vi "DAC_example.vi"() -> ()   [LabVIEW 2009]
panel:
  out "ACV Result":dbl[](array[numeric]) format="%.2e"
  out "Frequency Result":dbl[](array[numeric]) format="%.2e"
  out "VISA/Instrument Errors":errorcluster
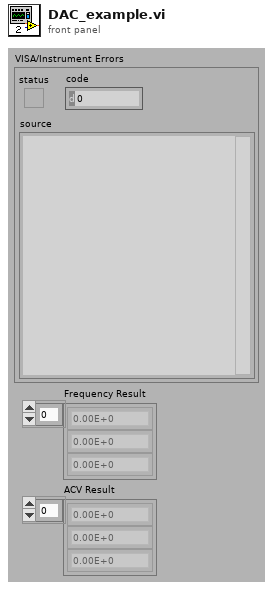
[diagram p1: front panel]
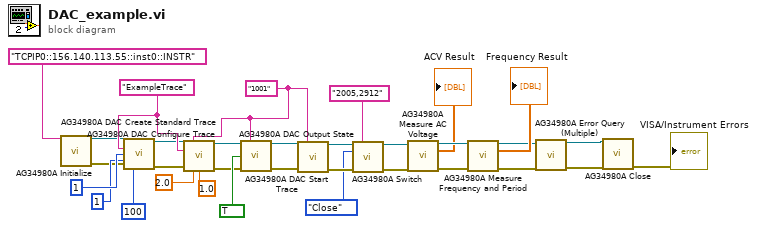
[diagram p0: block diagram]
diagram:
  w17 = "1001"
  w26 = "ExampleTrace"
  n1 = call "AG34980A Initialize.vi"("VISA resource name"="TCPIP0::156.140.113.55::inst0::INSTR") -> ("VISA session"=w25:refnum<visa-resource-name>, "error out"=w24:errorcluster)  [unwired: 13 in]
  n2 = call "AG34980A DAC Create Standard Trace.vi"("VISA resource name"=w25, "Trace Name"=w26, "Slot (1)"=1, "Trace Type"=1, "error in (no error)"=w24, "Num Points (1000)"=100) -> ("VISA resource name out"=w23:refnum<visa-resource-name>, "error out"=w22:errorcluster)  [unwired: 8 in]
  n3 = call "AG34980A DAC Configure Trace.vi"("VISA resource name"=w23, "Channel List"=w17, "Trace Name"=w26, "error in (no error)"=w22, "Gain (1)"=2.0, "Offset (0)"=1.0) -> ("VISA resource name out"=w21:refnum<visa-resource-name>, "error out"=w20:errorcluster)  [unwired: 8 in]
  n4 = call "AG34980A DAC Output State.vi"("VISA resource name"=w21, "Channel List"=w17, "Output State (F:Off)"=TRUE, "error in (no error)"=w20) -> ("VISA resource name out"=w19:refnum<visa-resource-name>, "error out"=w18:errorcluster)  [unwired: 10 in]
  n5 = call "AG34980A DAC Start Trace.vi"("VISA resource name"=w19, "Channel List"=w17, "error in (no error)"=w18) -> ("VISA resource name out"=w8:refnum<visa-resource-name>, "error out"=w7:errorcluster)  [unwired: 11 in]
  n6 = call "AG34980A Switch.vi"("VISA resource name"=w8, "Channel List"="2005,2912", "Open/Close (0:Close)"=enum16{"Close", "Open"}."Close", "error in (no error)"=w7) -> ("VISA resource name out"=w6:refnum<visa-resource-name>, "error out"=w5:errorcluster)  [unwired: 9 in, 1 out]
  n7 = call "AG34980A Measure AC Voltage.vi"("VISA resource name"=w6, "error in (no error)"=w5) -> ("VISA resource name out"=w13:refnum<visa-resource-name>, "Output Array"=→"ACV Result":dbl[], "error out"=w14:errorcluster)  [unwired: 11 in]
  n8 = call "AG34980A Measure Frequency and Period.vi"("VISA resource name"=w13, "error in (no error)"=w14) -> ("VISA resource name out"=w10:refnum<visa-resource-name>, "Output Array"=→"Frequency Result":dbl[], "error out"=w9:errorcluster)  [unwired: 11 in]
  n9 = call "AG34980A Error Query (Multiple).vi"("VISA resource name"=w10, "error in (no error)"=w9) -> ("VISA resource name out"=w15:refnum<visa-resource-name>, "error out"=w16:errorcluster)  [unwired: 10 in, 2 out]
  n10 = call "AG34980A Close.vi"("VISA resource name"=w15, "error in (no error)"=w16) -> ("error out"=→"VISA/Instrument Errors":errorcluster)  [unwired: 13 in]
